vi "习题7.2.vi"() -> ()   [LabVIEW 2017]
panel:
  out "波形图":dbl[][](graph)
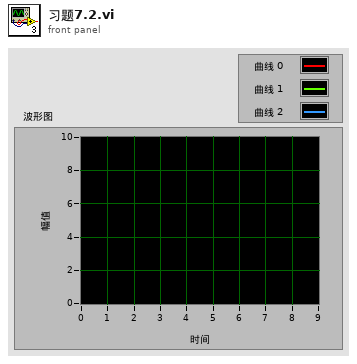
[diagram p1: front panel]
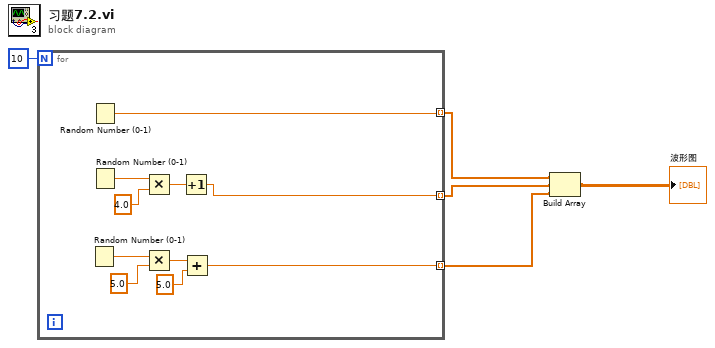
[diagram p0: block diagram]
diagram:
  n1 = for {
    N: 10 -> [_]
    tunnel: [w8] -> w4 mode=indexing
    tunnel: [w7] -> w3 mode=indexing
    tunnel: [w6] -> w2 mode=indexing
    n2 = Random Number (0-1)() -> (number: 0 to 1=w12:dbl)
    n3 = Random Number (0-1)() -> (number: 0 to 1=w8:dbl)
    n4 = Random Number (0-1)() -> (number: 0 to 1=w15:dbl)
    n5 = Multiply(x=w15, y=4.0) -> (x*y=w13:dbl)
    n6 = Multiply(x=w12, y=5.0) -> (x*y=w10:dbl)
    n7 = Increment(x=w13) -> (x+1=w7:dbl)
    n8 = Add(x=w10, y=5.0) -> (x+y=w6:dbl)
  }
  n9 = Build Array(w4, w3, w2) -> (→"波形图":dbl[][])
